vi "requiredCN0.vi"(2 "Channel Bandwith (MHz)":dbl, 3 "Eb/N0 required (dB)":dbl format="%#_13g", 4 "Bit rate (bits/s)":dbl) -> (0 "C/N required (dB)":dbl, 1 "C/N0 required (dB)":dbl)   [LabVIEW 2015]
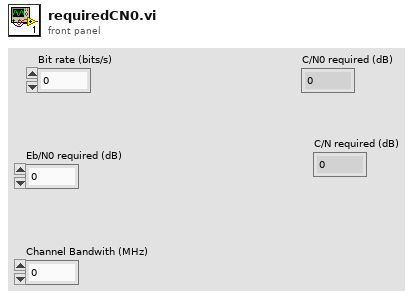
[diagram p1: front panel]
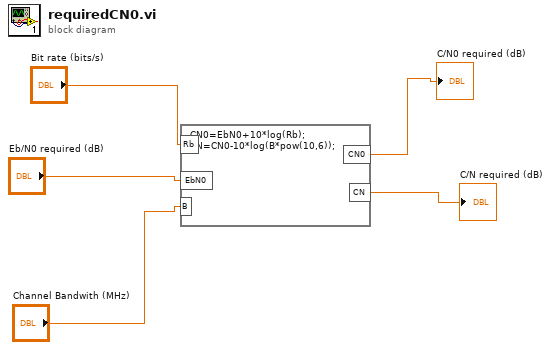
[diagram p0: block diagram]
diagram:
  n1 = formula code="CN0=EbN0+10*log(Rb);\nCN=CN0-10*log(B*pow(10,6));"("EbN0"="Eb/N0 required (dB)", "Rb"="Bit rate (bits/s)", "B"="Channel Bandwith (MHz)") -> ("CN0"=→"C/N0 required (dB)":dbl, "CN"=→"C/N required (dB)":dbl)
